vi "Stop Lock-In Path.vi"(7 "instance":i32, 8 "error in":errorcluster, 11 "fpga session in":refnum<k20>) -> (0 "error out":errorcluster, 3 "fpga session out":refnum<k20>)   [LabVIEW 2018, in "Lock-In Amplifier Example Host.lvlib"]
uses:
  Lock-In Amplifier Example Host.lvlib
  fpga type.ctl
  <vilib>/Utility/error.llb/Error Cluster From Error Code.vi
  <vilib>/rvi/errors/niLvFpgaAdjustHostInterfaceError.vi
  <vilib>/rvi/interface/nirviReadWriteControl/nirviReadWriteControl.xnode
  NiFpgaLv.dll
  <vilib>/rvi/interface/Simulation/niFpgaSimulationCallBeginRW.vi
  <instrlib>/_niInstr/Streaming/v1/Host/niInstr Streaming v1 Host.lvlib
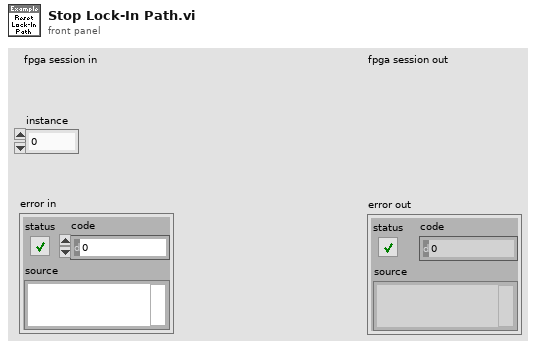
[diagram p1: front panel]
types:
  T1 = typedef "Lock-In Amplifier Example Host.lvlib/fpga type.ctl" = refnum<k20>
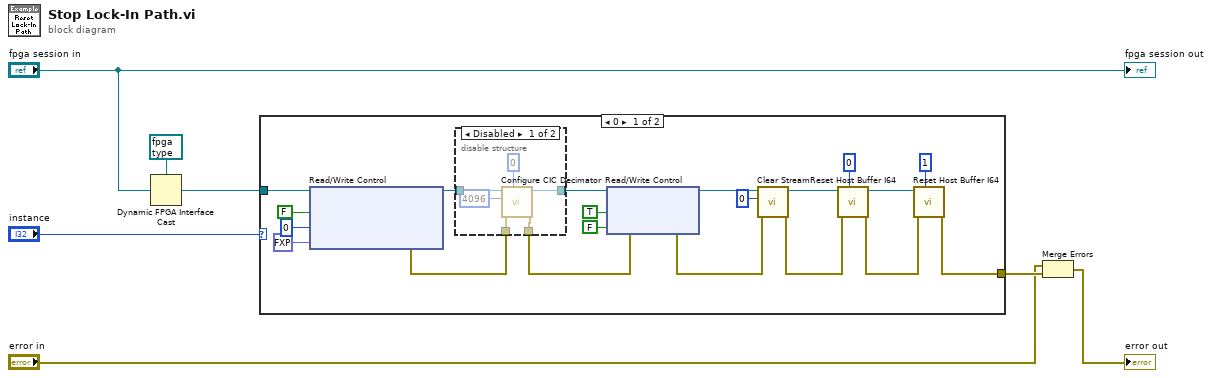
[diagram p0: block diagram]
diagram:
  n1 = Dynamic FPGA Interface Cast(Session In=T1 refnum ("fpga type"), Type="fpga session in") -> (Session Out=w5:T1)
  n2 = case shown="0" "instance" {
    tunnel: w5 -> [w27 _]
    tunnel: [w10 _] -> w3
    frame 0 {
      n3 = xnode "Read/Write Control"("FPGA VI Reference In"=w27, "lock-in.enable 0"=FALSE, "lock-in.carrier select 0"=0, "lock-in.carrier 0"=fxp<+/-,48,0> 0.0) -> ("FPGA VI Reference Out"=w23:T1, "error out"=w22:errorcluster)  [unwired: 1 in]
      n4 = disable-structure shown="Disabled" {
        disable-tunnel: w23 -> [w33 w35]
        disable-tunnel: w22 -> [w31 w34]
        disable-tunnel: [w29 w35] -> w21
        disable-tunnel: [w28 w34] -> w20
        frame Disabled {
          n5 = call "Configure CIC Decimator.vi"("index"=0, "error in"=w31, "decimation"=4096, "fpga session in"=w33) -> ("error out"=w28:errorcluster, "fpga session out"=w29:T1)  [unwired: 6 in]
        }
        frame Enabled {
        }
      }
      n6 = xnode "Read/Write Control"("FPGA VI Reference In"=w21, "error in"=w20, "lock-in.reset 0"=TRUE, "lock-in.reset 0"=FALSE ("lock-in.reset 1")) -> ("FPGA VI Reference Out"=w17:T1, "error out"=w16:errorcluster)
      n7 = call <instrlib>:"Clear Stream.vi"("error in (no error)"=w16, "stream index"=0, "refnum in"=w17) -> ("error out"=w13:errorcluster, "refnum out"=w14:T1)  [unwired: 7 in]
      n8 = call "Reset Host Buffer I64.vi"("index"=0, "error in"=w13, "fpga session in"=w14) -> ("error out"=w11:errorcluster, "fpga session out"=w12:T1)  [unwired: 7 in]
      n9 = call "Reset Host Buffer I64.vi"("index"=1, "error in"=w11, "fpga session in"=w12) -> ("error out"=w10:errorcluster)  [unwired: 7 in, 1 out]
    }
    frame Default {
    }
  }
  n10 = Merge Errors("error in", w3) -> (→"error out":errorcluster)
  "fpga session out" <- "fpga session in"
